vi "initialize_code.vi"() -> ()   [LabVIEW 2020]
panel:
  in  "VISA resource name":refnum<visa-resource-name>="USB0::0x0471::0x2515::482A16001::INSTR"
  in  "delay before read (ms)":u32=500
  out "error out 2":errorcluster
  out "read buffer":string
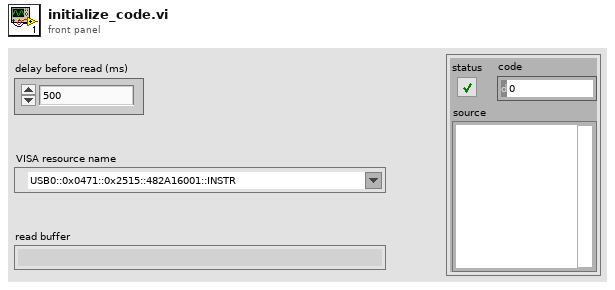
[diagram p1: front panel]
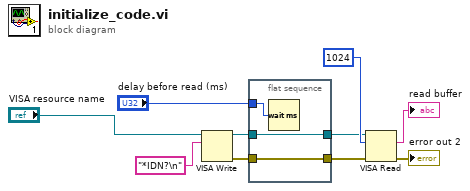
[diagram p0: block diagram]
diagram:
  n1 = VISA Write(VISA resource name="VISA resource name", write buffer="*IDN?\n") -> (VISA resource name out=w5:refnum<visa-resource-name>, error out=w4:errorcluster)  [unwired: 1 in, 1 out]
  n2 = flat-sequence {
    tunnel: w4 -> [w12]
    tunnel: [w12] -> w2
    tunnel: w5 -> [w11]
    tunnel: [w11] -> w3
    tunnel: "delay before read (ms)" -> [w13]
    frame #0 {
      n3 = Wait (ms)(milliseconds to wait=w13) -> ()  [unwired: 1 out]
    }
  }
  n4 = VISA Read(VISA resource name=w3, byte count=u32 1024, error in (no error)=w2) -> (read buffer=→"read buffer":string, error out=→"error out 2":errorcluster)  [unwired: 2 out]
